vi "ryTimer Status.vi"(8 "error in (no error)":errorcluster, 11 "Timer in":refnum<class "ryTimer.lvclass">) -> (0 "error out":errorcluster, 1 "Time Left (ms) [-1=Unknown]":i32, 2 "Is Running?":bool, 3 "Timer out":refnum<class "ryTimer.lvclass">, 4 "Wait Time (ms)":u32, 6 "Last Ticks (ms)":u32)   [LabVIEW 2020, in "ryTimer.lvclass"]
doc: "Returns the timer status. <b>Is Running?</b> returns True if the timer is running and the <b>Wait Time (ms)</b> is greater than zero. The <b>Time Left (ms)</b> is the time remaining until the next emit and <b>Last Ticks (ms)</b> is the internal tick counter value used to recalculate the daemon thread rate."
uses:
  ryTimer.lvclass
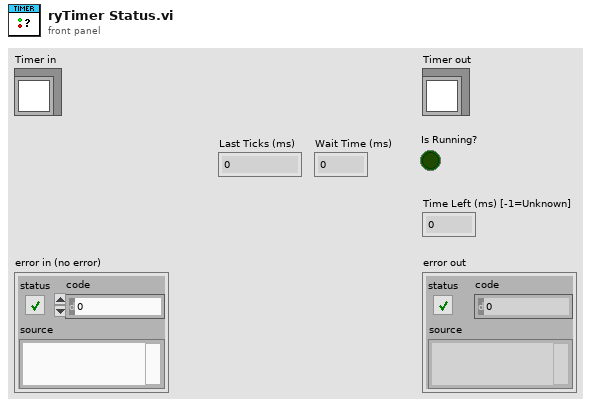
[diagram p1: front panel]
types:
  T1 = typedef "ryTimer.lvclass/ryTimer Properties.ctl" = cluster{"Wait Time (ms)":u32, "Is Running":bool, "Last Ticks":u32, "Emit":refnum<queue>}
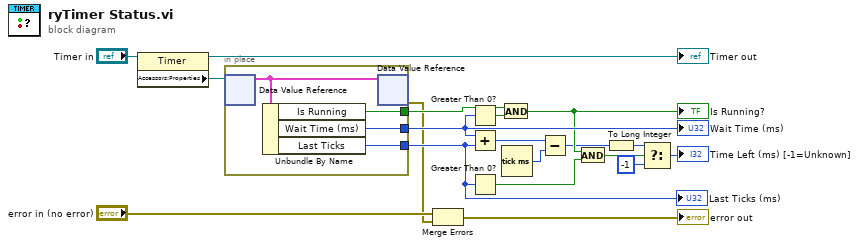
[diagram p0: block diagram]
diagram:
  n1 = property class="Timer"(reference="Timer in") -> (reference out=→"Timer out":refnum<class "ryTimer.lvclass">, "Accessors:Properties"=w2:refnum<data-value>)  [unwired: 1 in, 1 out]
  n2 = in-place {
    in-place-border: [w23] -> w17
    in-place-border: [w22] -> w12
    in-place-border: [w20] -> w10
    n3 = in-place-dvr #1(w2) -> (w21:T1)  [unwired: 1 out]
    n4 = Unbundle By Name(w21) -> ("Is Running"=w22:bool, "Wait Time (ms)"=w23:u32, "Last Ticks"=w20:u32)
    n5 = in-place-dvr #1(w21) -> (w4:errorcluster)  [unwired: 1 out]
  }
  "Wait Time (ms)" <- w17
  "Last Ticks (ms)" <- w10
  n6 = Merge Errors("error in (no error)", w4) -> (→"error out":errorcluster)
  n7 = Greater Than 0?(x=w17) -> (x > 0?=w19:bool)
  n8 = Add(x=w17, y=w10) -> (x+y=w13:u32)
  n9 = Greater Than 0?(x=w10) -> (x > 0?=w7:bool)
  n10 = And(x=w12, y=w19) -> (x .and. y?=w16:bool)
  "Is Running?" <- w16
  n11 = Tick Count (ms)() -> (millisecond timer value=w18:u32)
  n12 = Subtract(x=w13, y=w18) -> (x-y=w11:u32)
  n13 = And(x=w16, y=w7) -> (x .and. y?=w8:bool)
  n14 = To Long Integer(number=w11) -> (32bit integer=w9:i32)
  n15 = Select(t=w9, s=w8, f=-1) -> (s? t:f=→"Time Left (ms) [-1=Unknown]":i32)
